vi "MDAQ_IndexInc.vi"(10 "Input Cluster":T1 {"CV"."Temperature Array" scale=0.0..100.0}) -> (2 "Output Cluster":T1 {"CV"."Temperature Array" scale=0.0..100.0})   [LabVIEW 2021]
uses:
  GUI_Def.ctl
  Mode_Enum.ctl
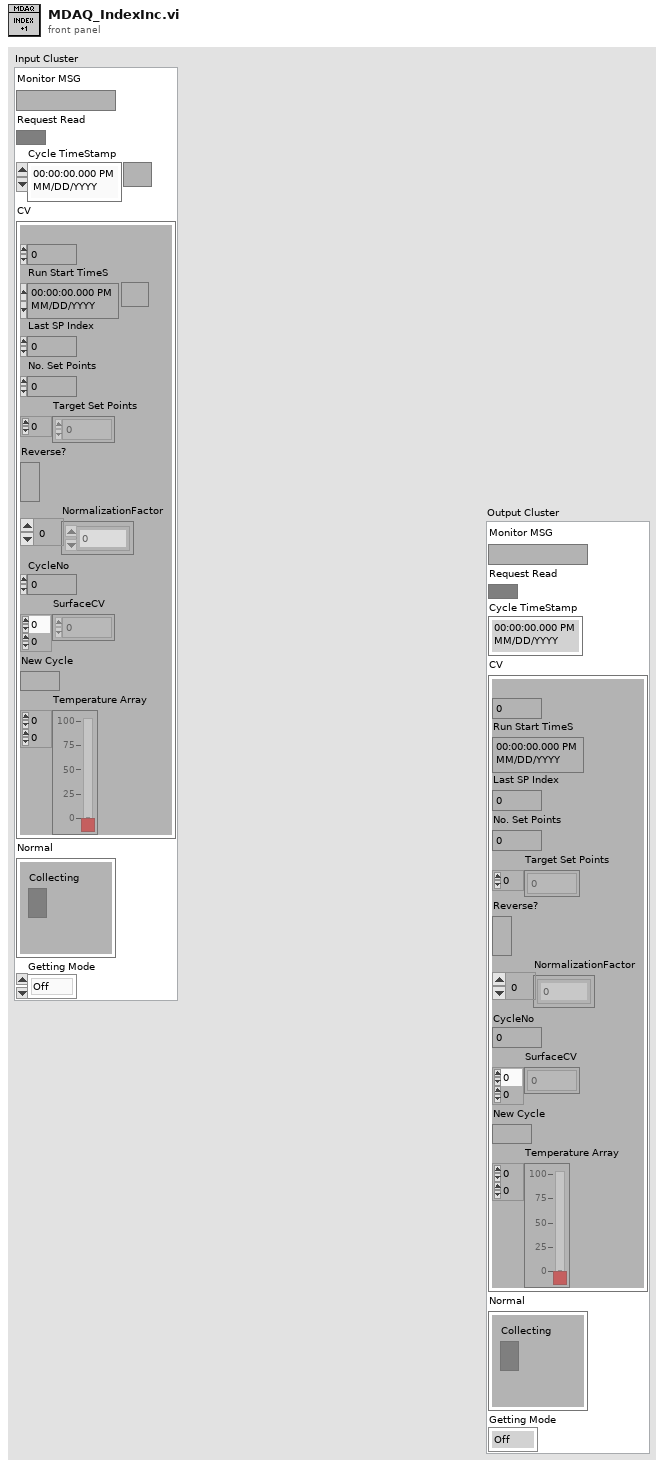
[diagram p1: front panel]
types:
  T1 = typedef "GUI_Def.ctl" = cluster{"Monitor MSG":string, "Request Read":bool, "Cycle TimeStamp":timestamp, "CV":cluster{"Set Point Index":u32, "Run Start TimeS":timestamp, "Last SP Index":u32, "No. Set Points":u32, "Target Set Points":i32[], "Reverse?":bool, "NormalizationFactor":i32[], "CycleNo":i32, "SurfaceCV":dbl[][], "New Cycle":bool, "Temperature Array":dbl[][]}, "Normal":cluster{"Collecting":bool}, "Getting Mode":T2}
  T2 = typedef "Mode_Enum.ctl" = enum16{"Off", "Normal", "CV+Temp", "CV"}
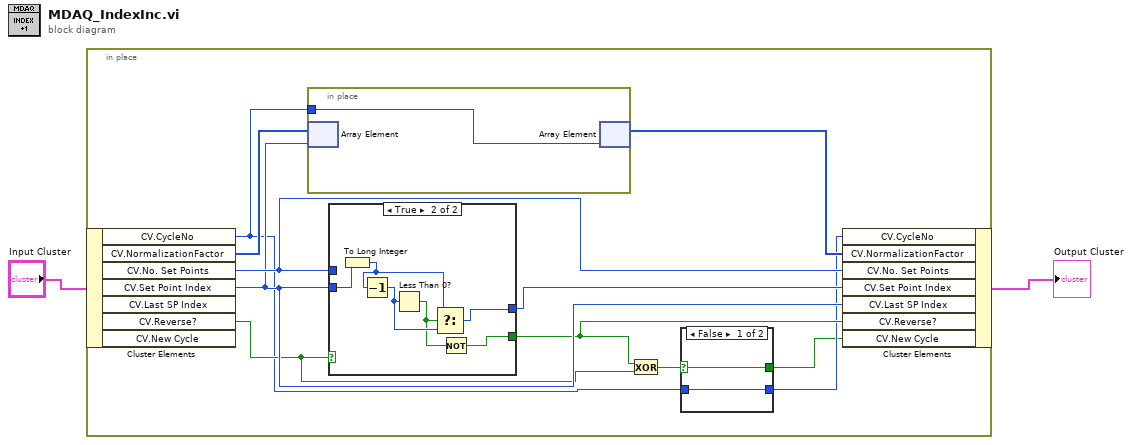
[diagram p0: block diagram]
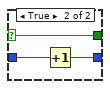
[diagram p2: hidden frame]
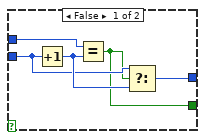
[diagram p3: hidden frame]
diagram:
  n1 = in-place {
    n2 = in-place-cluster #1("Input Cluster") -> ("CV.CycleNo"=w4:i32, "CV.NormalizationFactor"=w11:i32[], "CV.No. Set Points"=w12:u32, "CV.Set Point Index"=w10:u32, "CV.Reverse?"=w8:bool)  [unwired: 2 out]
    n3 = in-place {
      in-place-border: w4 -> [w19]
      n4 = in-place-array #2(w11, w10) -> ()  [unwired: 1 out]
      n5 = in-place-array #2(w19) -> (w9:i32[])  [unwired: 1 out]
    }
    n6 = case shown="True" w8 {
      tunnel: w10 -> [w22 w26]
      tunnel: w12 -> [w24 _]
      tunnel: [w21 w29] -> w13
      tunnel: [w20 w28] -> w7
      frame False {
        n7 = Increment(x=w22) -> (x+1=w23:u32)
        n8 = Equal?(x=w24, y=w23) -> (x = y?=w20:bool)
        n9 = Select(t=w22, s=w20, f=w23) -> (s? t:f=w21:u32)
      }
      frame True {
        n10 = To Long Integer(number=w26) -> (32bit integer=w25:i32)
        n11 = Decrement(x=w25) -> (x-1=w30:i32)
        n12 = Less Than 0?(x=w30) -> (x < 0?=w27:bool)
        n13 = Select(t=w25, s=w27, f=w30) -> (s? t:f=w29:i32)
        n14 = Not(x=w27) -> (.not. x?=w28:bool)
      }
    }
    n15 = Exclusive Or(1:w8, 2:w7) -> (0:w6:bool)
    n16 = case shown="False" w6 {
      selector: w6 -> [w14 w16]
      tunnel: w4 -> [w15 w18]
      tunnel: [w15 w17] -> w5
      tunnel: [w14 w16] -> w3
      frame False {
      }
      frame True {
        n17 = Increment(x=w18) -> (x+1=w17:i32)
      }
    }
    n18 = in-place-cluster #1("CV.CycleNo"=w5, "CV.NormalizationFactor"=w9, "CV.No. Set Points"=w12, "CV.Set Point Index"=w13, "CV.Last SP Index"=w10, "CV.Reverse?"=w7, "CV.New Cycle"=w3) -> (→"Output Cluster":T1)
  }
